vi "Secure-Release Region.vi"(7 "Action":enum16{"Secure", "Release"}(ring), 8 "error in (no error)":errorcluster, 10 "Control In":T1={"I-O.lvclass"=refnum, "Motion.lvclass"=refnum, "Dispenser.lvclass"=refnum}, 11 "Fixture in":refnum<class "Fixture.lvclass">) -> (0 "error out":errorcluster, 2 "Control Out":T1, 3 "Fixture out":refnum<class "Fixture.lvclass">)   [LabVIEW 2016, in "Fixture.lvclass"]
uses:
  Fixture.lvclass
  Controller/Controllers.ctl
  Controller/I-O/I-O.lvclass
  Controller/Motion/A3200/A3200.lvclass
  Controller/Dispenser/Dispenser.lvclass
  Controller/Motion/Motion.lvclass
  Fixture.lvclass/Fixture.ctl
  Controller/Controller.lvclass
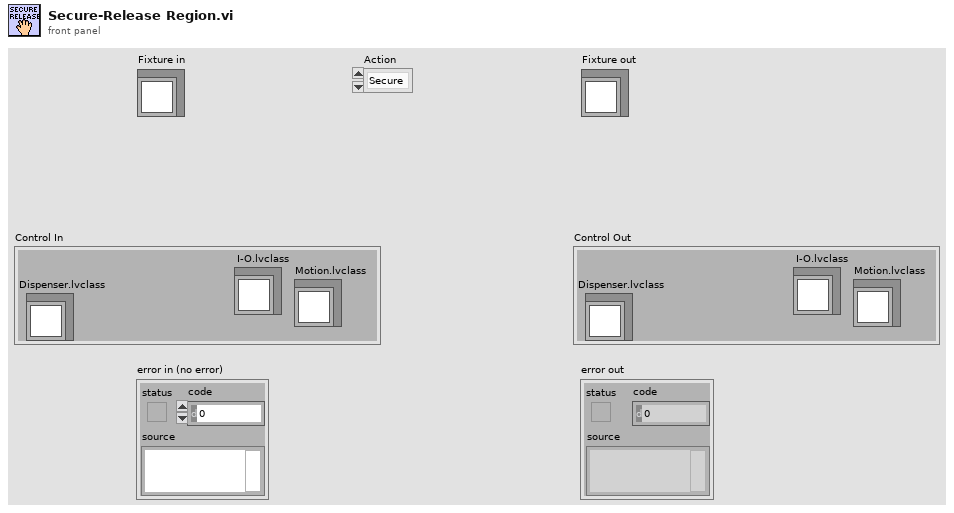
[diagram p1: front panel]
types:
  T1 = typedef "Controller.lvclass/Controllers.ctl" = cluster{"I-O.lvclass":refnum<class "I-O.lvclass">, "Motion.lvclass":refnum<class "Motion.lvclass">, "Dispenser.lvclass":refnum<class "Dispenser.lvclass">}
  T2 = typedef "I-O.lvclass/Pin Map.ctl" = cluster{"Region Valves":i32[], "Extra Valves":dbl[][][], "Tool Primary Valve":i32, "Tool Secondary Valve":i32, "Region Sensors":i32[], "Extra Sensors":dbl[][][], "Tool Primary Sensor":dbl, "Tool Secondary Sensor":dbl, "Compression Sensor":dbl, "5V":i32}
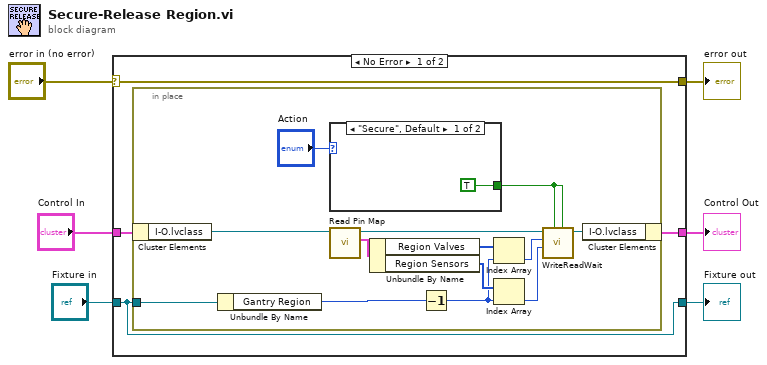
[diagram p0: block diagram]
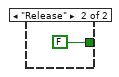
[diagram p2: hidden frame]
diagram:
  n1 = case shown="No Error" "error in (no error)" {
    selector: "error in (no error)" -> [w10 w28]
    tunnel: [w10 w28] -> w5
    tunnel: [w8 w27] -> w3
    tunnel: "Fixture in" -> [w8 w27]
    tunnel: "Control In" -> [w9 w26]
    tunnel: [w7 w26] -> w1
    frame No Error {
      n2 = in-place {
        in-place-border: w8 -> [w22]
        n3 = in-place-cluster #1(w9) -> ("I-O.lvclass"=w19:refnum<class "I-O.lvclass">)
        n4 = Unbundle By Name(w22) -> ("Gantry Region"=w16:i32)
        n5 = case shown="\"Secure\", Default" "Action" {
          tunnel: [TRUE FALSE] -> w20
          frame "Secure", Default {
          }
          frame "Release" {
          }
        }
        n6 = call-dynamic "Read Pin Map.vi"("I-O in"=w19) -> ("Pin Map 2"=w18:T2, "I-O out"=w17:refnum<class "I-O.lvclass">)  [unwired: 8 in, 1 out]
        n7 = Unbundle By Name(w18) -> ("Region Valves"=w15:i32[], "Region Sensors"=w14:i32[])
        n8 = Decrement(x=w16) -> (x-1=w11:i32)
        n9 = Index Array(array=w15, index=w11) -> (element=w13:i32)
        n10 = Index Array(array=w14, index=w11) -> (element=w12:i32)
        n11 = call "WriteReadWait.vi"("Read Value"=w20, "Write Value"=w20, "Read"=w12, "Write"=w13, "I-O in"=w17) -> ("I-O out"=w23:refnum<class "I-O.lvclass">)  [unwired: 5 in, 1 out]
        n12 = in-place-cluster #1("I-O.lvclass"=w23) -> (w7:T1)
      }
    }
    frame Error {
    }
  }
  "error out" <- w5
  "Fixture out" <- w3
  "Control Out" <- w1
